vi "Set State.vi"(8 "error in (no error)":errorcluster, 10 "state":T1, 11 "output_actor_errorneous in":refnum<class "Output Actor Hardware.lvclass">) -> (0 "error out":errorcluster, 3 "output_actor_errorneous out":refnum<class "Output Actor Hardware.lvclass">)   [LabVIEW 2015, in "Output Actor Hardware.lvclass"]
uses:
  Output Actor Hardware.lvclass
  state.ctl
  Output Actor Hardware.lvclass/Output Actor Hardware.ctl
  output actor/Output Actor.lvclass
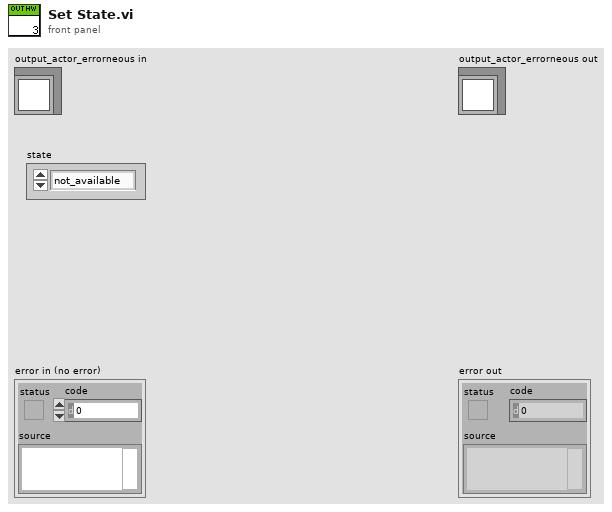
[diagram p1: front panel]
types:
  T1 = typedef "Output Actor Hardware.lvclass/state.ctl" = enum16{"not_available", "not_initialized", "ok"}
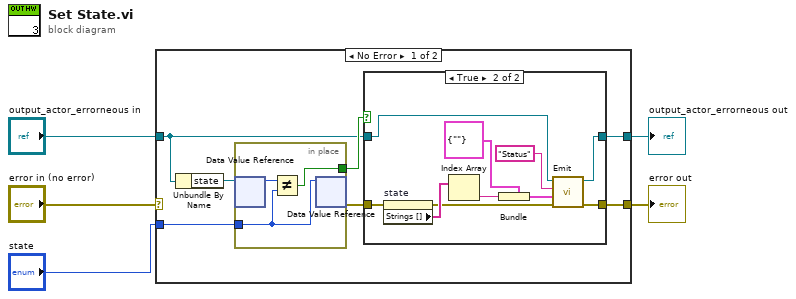
[diagram p0: block diagram]
diagram:
  n1 = case shown="No Error" "error in (no error)" {
    selector: "error in (no error)" -> [_ w29]
    tunnel: [w7 w29] -> w4
    tunnel: [w8 w28] -> w2
    tunnel: "output_actor_errorneous in" -> [w9 w28]
    tunnel: "state" -> [w11 _]
    frame No Error {
      n2 = Unbundle By Name(w9) -> ("state"=w12:refnum<data-value>)
      n3 = in-place {
        in-place-border: w11 -> [w26]
        in-place-border: [w25] -> w10
        n4 = in-place-dvr #1(w12) -> (w27:T1)  [unwired: 1 out]
        n5 = Not Equal?(x=w27, y=w26) -> (x != y?=w25:bool)
        n6 = in-place-dvr #1(w26) -> (w6:errorcluster)  [unwired: 1 out]
      }
      n7 = case shown="True" w10 {
        tunnel: [w13 w18] -> w7
        tunnel: [w14 w17] -> w8
        tunnel: w9 -> [w14 w16]
        tunnel: w6 -> [w13 w15]
        frame False {
        }
        frame True {
          n8 = property on="state" class="Enum (strict)"(error in=w15) -> (error out=w19:errorcluster, "Strings []"=w20:string[])  [unwired: 1 in, 1 out]
          n9 = Index Array(array=w20) -> (element=w23:string)  [unwired: 1 in]
          n10 = Bundle(cluster=cluster{"Status":string} {"Status"=""}, "Status"=w23) -> (w24:cluster{"Status":string})
          n11 = call "Emit.vi"("error in (no error)"=w19, "parameter"=w24, "function"="Status", "output_actor in"=w16) -> ("error out"=w18:errorcluster, "output_actor out"=w17:refnum<class "Output Actor Hardware.lvclass">)  [unwired: 6 in]
        }
      }
    }
    frame Error {
    }
  }
  "error out" <- w4
  "output_actor_errorneous out" <- w2
